vi "ZeroMQ_ReqRep_generic.vi"() -> ()   [LabVIEW 2018]
uses:
  <vilib>/addons/zeromq/socket_type.ctl
  <vilib>/addons/zeromq/socket_options.ctl
  <vilib>/addons/zeromq/zeromq.lvlib
  <vilib>/addons/zeromq/zmq_socket.lvclass
  <vilib>/addons/zeromq/zmq_context.lvclass
panel:
  out "reply":string
  in  "stop 3":bool
  out "command":string
  out "error out 3":errorcluster
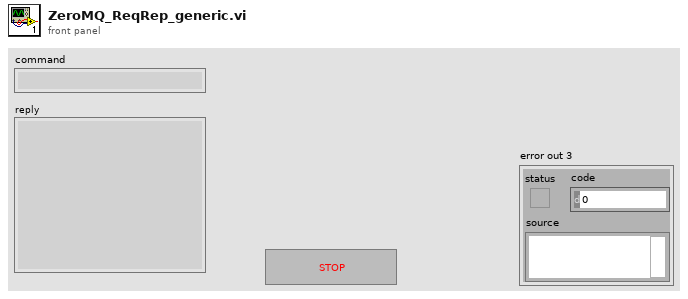
[diagram p1: front panel]
types:
  T1 = cluster{"ID":u32, "Address":string, "Service Name 1":string, "Service Name 2":string, "queue TX":refnum<queue>, "queue RX":refnum<queue>, "Port 1":u32, "Port 2":u32}
  T2 = typedef "zeromq.lvlib/socket_options.ctl" = enum8{"NONE", "ZMQ_HWM", "<2>", "ZMQ_SWAP", "ZMQ_AFFINITY", "ZMQ_ROUTING_ID", "ZMQ_SUBSCRIBE", "ZMQ_UNSUBSCRIBE", "ZMQ_RATE", "ZMQ_RECOVERY_IVL", "ZMQ_MCAST_LOOP", "ZMQ_SNDBUF", "ZMQ_RCVBUF", "ZMQ_RCVMORE", "ZMQ_FD", "ZMQ_EVENTS", "ZMQ_TYPE", "ZMQ_LINGER", "ZMQ_RECONNECT_IVL", "ZMQ_BACKLOG", "ZMQ_RECOVERY_IVL_MSEC", "ZMQ_RECONNECT_IVL_MAX", "ZMQ_MAXMSGSIZE", "ZMQ_SNDHWM", "ZMQ_RCVHWM", "ZMQ_MULTICAST_HOPS", "<26>", "ZMQ_RCVTIMEO", "ZMQ_SNDTIMEO", "<29>", "<30>", "ZMQ_IPV4ONLY", "ZMQ_LAST_ENDPOINT", "ZMQ_ROUTER_MANDATORY", "ZMQ_TCP_KEEPALIVE", "ZMQ_TCP_KEEPALIVE_CNT", "ZMQ_TCP_KEEPALIVE_IDLE", "ZMQ_TCP_KEEPALIVE_INTVL", "ZMQ_TCP_ACCEPT_FILTER", "ZMQ_IMMEDIATE", "ZMQ_XPUB_VERBOSE", "ZMQ_ROUTER_RAW", "ZMQ_IPV6", "ZMQ_MECHANISM", "ZMQ_PLAIN_SERVER", "ZMQ_PLAIN_USERNAME", "ZMQ_PLAIN_PASSWORD", "ZMQ_CURVE_SERVER", "ZMQ_CURVE_PUBLICKEY", "ZMQ_CURVE_SECRETKEY", "ZMQ_CURVE_SERVERKEY", "ZMQ_PROBE_ROUTER", "ZMQ_REQ_CORRELATE", "ZMQ_REQ_RELAXED", "ZMQ_CONFLATE", "ZMQ_ZAP_DOMAIN", "ZMQ_ROUTER_HANDOVER", "ZMQ_TOS", "ZMQ_IPC_FILTER_PID", "ZMQ_IPC_FILTER_UID", "ZMQ_IPC_FILTER_GID", "ZMQ_CONNECT_ROUTING_ID", "ZMQ_GSSAPI_SERVER", "ZMQ_GSSAPI_PRINCIPAL", "ZMQ_GSSAPI_SERVICE_PRINCIPAL", "ZMQ_GSSAPI_PLAINTEXT", "ZMQ_HANDSHAKE_IVL", "<67>", "ZMQ_SOCKS_PROXY", "ZMQ_XPUB_NODROP", "ZMQ_BLOCKY", "ZMQ_XPUB_MANUAL", "ZMQ_XPUB_WELCOME_MSG", "ZMQ_STREAM_NOTIFY", "ZMQ_INVERT_MATCHING", "ZMQ_HEARTBEAT_IVL", "ZMQ_HEARTBEAT_TTL", "ZMQ_HEARTBEAT_TIMEOUT", "ZMQ_XPUB_VERBOSER", "ZMQ_CONNECT_TIMEOUT", "ZMQ_TCP_MAXRT", "ZMQ_THREAD_SAFE", "<82>", "<83>", "ZMQ_MULTICAST_MAXTPDU", "ZMQ_VMCI_BUFFER_SIZE", "ZMQ_VMCI_BUFFER_MIN_SIZE", "ZMQ_VMCI_BUFFER_MAX_SIZE", "ZMQ_VMCI_CONNECT_TIMEOUT", "ZMQ_USE_FD", "ZMQ_GSSAPI_PRINCIPAL_NAMETYPE", "ZMQ_GSSAPI_SERVICE_PRINCIPAL_NAMETYPE", "ZMQ_BINDTODEVICE", "ZMQ_ZAP_ENFORCE_DOMAIN", "ZMQ_LOOPBACK_FASTPATH", "ZMQ_METADATA", "ZMQ_MULTICAST_LOOP", "ZMQ_ROUTER_NOTIFY"}
  T3 = typedef "zeromq.lvlib/socket_type.ctl" = enum8{"ZMQ_PAIR", "ZMQ_PUB", "ZMQ_SUB", "ZMQ_REQ", "ZMQ_REP", "ZMQ_DEALER", "ZMQ_ROUTER", "ZMQ_PULL", "ZMQ_PUSH", "ZMQ_XPUB", "ZMQ_XSUB", "ZMQ_STREAM", "ZMQ_SERVER", "ZMQ_CLIENT", "ZMQ_RADIO", "ZMQ_DISH", "ZMQ_GATHER", "ZMQ_SCATTER", "ZMQ_DGRAM"}
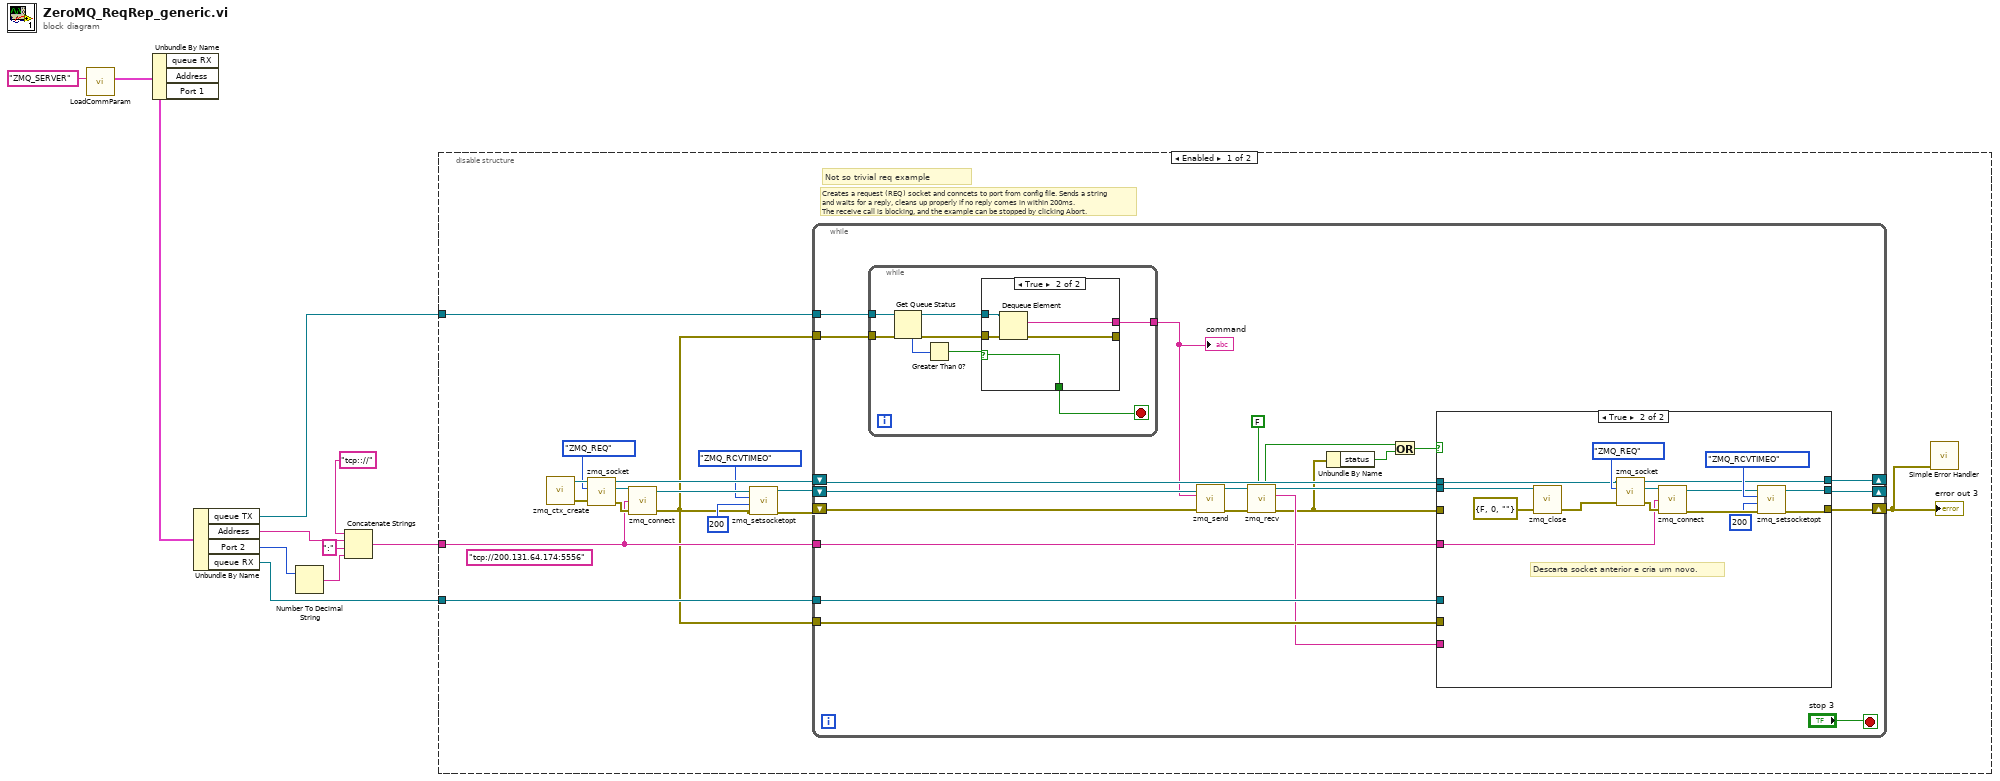
[diagram p0: block diagram]
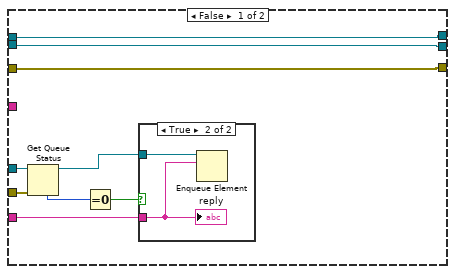
[diagram p2: hidden frame]
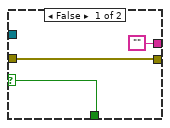
[diagram p4: hidden frame]
diagram:
  n1 = call "LoadCommParam.vi"("section name"="ZMQ_SERVER") -> ("output cluster"=w9:T1)  [unwired: 10 in]
  n2 = Unbundle By Name(w9) -> ()  [unwired: 3 out]
  n3 = Unbundle By Name(w9) -> ("queue TX"=w8:refnum<queue>, "Address"=w6:string, "Port 2"=w4:u32, "queue RX"=w1:refnum<queue>)
  n4 = Number To Decimal String(number=w4) -> (decimal integer string=w3:string)  [unwired: 1 in]
  n5 = Concatenate Strings("tcp:://" ("string"), w6, ":" ("string"), w3) -> (w2:string)
  n6 = disable-structure shown="Enabled" {
    disable-tunnel: w8 -> [w19 _]
    disable-tunnel: w2 -> [w18 _]
    disable-tunnel: w1 -> [w12 _]
    frame Enabled {
      (unwired) "tcp://200.131.64.174:5556" ("endpoint")
      # "Creates a request (REQ) socket and conncets to port from config file. Sends a string and waits for a reply, cleans up properly if no reply comes in within 200ms.\nThe receive call is blocking, and the example can be stopped by clicking Abort."
      # "Not so trivial req example"
      n7 = call <vilib>:"zmq_ctx_create.vi"() -> ("error out"=w25:errorcluster, "context out"=w22:refnum<class "zmq_context.lvclass">)  [unwired: 4 in]
      n8 = call <vilib>:"zmq_socket.vi"("error in"=w25, "socket type"=socket_type."ZMQ_REQ", "context in"=w22) -> ("error out"=w23:errorcluster, "socket out"=w24:refnum<class "zmq_socket.lvclass">, "context out"=w20:refnum<class "zmq_context.lvclass">)  [unwired: 2 in]
      n9 = call <vilib>:"zmq_connect.vi"("error in"=w23, "endpoint"=w18, "socket in"=w24) -> ("error out"=w11:errorcluster, "socket out"=w17:refnum<class "zmq_socket.lvclass">)  [unwired: 1 in]
      n10 = call <vilib>:"zmq_setsocketopt.vi"("error in"=w11, "value"=200 ("max queue size (-1, unlimited)"), "option"=socket_options."ZMQ_RCVTIMEO", "socket in"=w17) -> ("error out"=w13:errorcluster, "socket out"=w16:refnum<class "zmq_socket.lvclass">)  [unwired: 2 in]
      n11 = while {
        tunnel: w19 -> [w46]
        tunnel: w11 -> [w45]
        tunnel: w12 -> [w44]
        tunnel: w11 -> [w43]
        shift-right: [w36] -> _
        shift-left: w20 -> [w38]
        shift-right: [w35] -> _
        shift-left: w16 -> [w39]
        shift-right: [w34] -> w26
        shift-left: w13 -> [w40]
        tunnel: w18 -> [w33]
        stop <- "stop 3" stop-if-true
        n12 = while {
          tunnel: w46 -> [w81]
          tunnel: w45 -> [w80]
          tunnel: [w76] -> w31
          stop <- w75 stop-if-true
          n13 = Get Queue Status(queue=w81, error in (no error)=w80) -> (queue out=w77:refnum<queue>, error out=w78:errorcluster, # elements in queue=w82:i32)  [unwired: 1 in, 5 out]
          n14 = Greater Than 0?(x=w82) -> (x > 0?=w79:bool)
          n15 = case shown="True" w79 {
            selector: w79 -> [w83 w86]
            tunnel: w78 -> [w85 w90]
            tunnel: w77 -> [_ w89]
            tunnel: [w85 w88] -> _
            tunnel: ["" w87] -> w76
            tunnel: [w83 w86] -> w75
            frame False {
            }
            frame True {
              n16 = Dequeue Element(queue=w89, error in (no error)=w90) -> (element=w87:string, error out=w88:errorcluster)  [unwired: 1 in, 2 out]
            }
          }
        }
        "command" <- w31
        n17 = call <vilib>:"zmq_send.vi"("error in"=w40, "data"=w31, "socket in"=w39) -> ("error out"=w47:errorcluster, "socket out"=w48:refnum<class "zmq_socket.lvclass">)  [unwired: 4 in]
        n18 = call <vilib>:"zmq_recv.vi"("no block? (F)"=FALSE, "error in"=w47, "socket in"=w48) -> ("error out"=w30:errorcluster, "data"=w42:string, "socket out"=w37:refnum<class "zmq_socket.lvclass">, "timeout?"=w28:bool)  [unwired: 2 in, 1 out]
        n19 = Unbundle By Name(w30) -> ("status"=w27:bool)
        n20 = Or(x=w28, y=w27) -> (x .or. y?=w29:bool)
        n21 = case shown="True" w29 {
          tunnel: w44 -> [w56 _]
          tunnel: w42 -> [w53 _]
          tunnel: w43 -> [w52 _]
          tunnel: w38 -> [w50 w62]
          tunnel: w30 -> [w49 _]
          tunnel: w37 -> [w51 w63]
          tunnel: [w50 w64] -> w36
          tunnel: [w51 w65] -> w35
          tunnel: [w49 w66] -> w34
          tunnel: w33 -> [_ w67]
          frame False {
            n22 = Get Queue Status(queue=w56, error in (no error)=w52) -> (queue out=w54:refnum<queue>, # elements in queue=w57:i32)  [unwired: 1 in, 6 out]
            n23 = Equal To 0?(x=w57) -> (x = 0?=w55:bool)
            n24 = case shown="True" w55 {
              tunnel: w54 -> [_ w59]
              tunnel: w53 -> [_ w58]
              frame False {
              }
              frame True {
                n25 = Enqueue Element(queue=w59, element=w58) -> ()  [unwired: 2 in, 3 out]
                "reply" <- w58
              }
            }
          }
          frame True {
            # "Descarta socket anterior e cria um novo."
            n26 = call <vilib>:"zmq_close.vi"("error in"=errorcluster {"status"=FALSE, "code"=0, "source"=""}, "socket"=w63) -> ("error out"=w60:errorcluster)  [unwired: 3 in]
            n27 = call <vilib>:"zmq_socket.vi"("error in"=w60, "socket type"=socket_type."ZMQ_REQ", "context in"=w62) -> ("error out"=w73:errorcluster, "socket out"=w74:refnum<class "zmq_socket.lvclass">, "context out"=w64:refnum<class "zmq_context.lvclass">)  [unwired: 2 in]
            n28 = call <vilib>:"zmq_connect.vi"("error in"=w73, "endpoint"=w67, "socket in"=w74) -> ("error out"=w69:errorcluster, "socket out"=w70:refnum<class "zmq_socket.lvclass">)  [unwired: 1 in]
            n29 = call <vilib>:"zmq_setsocketopt.vi"("error in"=w69, "value"=200 ("max queue size (-1, unlimited)"), "option"=socket_options."ZMQ_RCVTIMEO", "socket in"=w70) -> ("error out"=w66:errorcluster, "socket out"=w65:refnum<class "zmq_socket.lvclass">)  [unwired: 2 in]
          }
        }
      }
      "error out 3" <- w26
      n30 = call <vilib>:"Simple Error Handler.vi"("error in (no error)"=w26) -> ()  [unwired: 4 in, 5 out]
    }
    frame Disabled {
    }
  }
